vi "Get All Paths.vi"(11 "error in":errorcluster) -> (4 "Log Folder":path, 6 "Settings Folder":path, 10 "Smart Guider App file":path, 15 "error out":errorcluster)   [LabVIEW 2014]
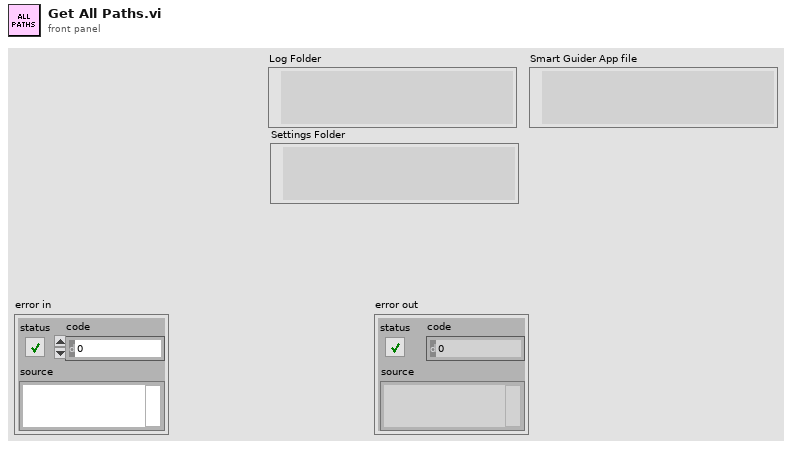
[diagram p1: front panel]
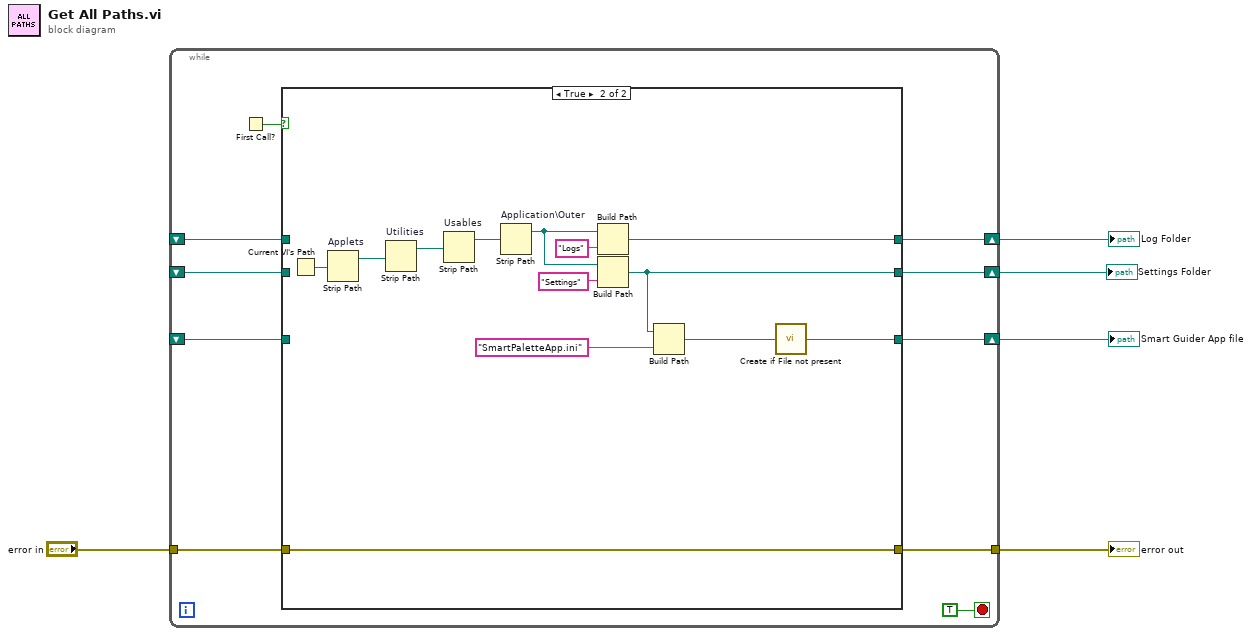
[diagram p0: block diagram]
diagram:
  n1 = while {
    tunnel: [w11] -> w3
    tunnel: "error in" -> [w10]
    shift-right: [w15] -> w5
    shift-left: _ -> [w9]
    shift-right: [w14] -> w4
    shift-left: _ -> [w8]
    shift-right: [w7] -> w1
    shift-left: _ -> [w6]
    stop <- TRUE stop-if-true
    n2 = First Call?() -> (First Call?: T/F=w12:bool)
    n3 = case shown="True" w12 {
      tunnel: [w18 w28] -> w15
      tunnel: [w17 w22] -> w14
      tunnel: [w19 w24] -> w11
      tunnel: w10 -> [w19 w24]
      tunnel: w9 -> [w18 _]
      tunnel: w8 -> [w17 _]
      tunnel: [w16 w20] -> w7
      tunnel: w6 -> [w16 _]
      frame False {
      }
      frame True {
        n4 = Current VI's Path() -> (path=w30:path)
        n5 = Strip Path "Applets"(path=w30) -> (stripped path=w32:path)  [unwired: 1 out]
        n6 = Strip Path "Utilities"(path=w32) -> (stripped path=w31:path)  [unwired: 1 out]
        n7 = Strip Path "Usables"(path=w31) -> (stripped path=w25:path)  [unwired: 1 out]
        n8 = Strip Path "Application\\Outer"(path=w25) -> (stripped path=w26:path)  [unwired: 1 out]
        n9 = Build Path(base path=w26, name or relative path="Logs") -> (appended path=w28:path)
        n10 = Build Path(base path=w26, name or relative path="Settings") -> (appended path=w22:path)
        n11 = Build Path(base path=w22, name or relative path="SmartPaletteApp.ini") -> (appended path=w21:path)
        n12 = call "Create if File not present.vi"("File in"=w21) -> ("File out"=w20:path)
      }
    }
  }
  "error out" <- w3
  "Log Folder" <- w5
  "Settings Folder" <- w4
  "Smart Guider App file" <- w1
